vi "Make String.vi"(8 "error in (no error)":errorcluster, 11 "Construct String Setup Cam in":refnum<class "Construct String Setup Cam.lvclass">) -> (0 "error out":errorcluster, 2 "Camera Setup":string, 3 "Construct String Setup Cam out":refnum<class "Construct String Setup Cam.lvclass">)   [LabVIEW 2018, in "Construct String Setup Cam.lvclass"]
doc: "Este VI faz a leitura da configuração da câmera e constrói uma string com as informações da configuração."
uses:
  Construct String Setup Cam.lvclass
  Construct String Setup Cam.lvclass/Construct String Setup Cam.ctl
panel:
  out "Camera Setup 2":T1
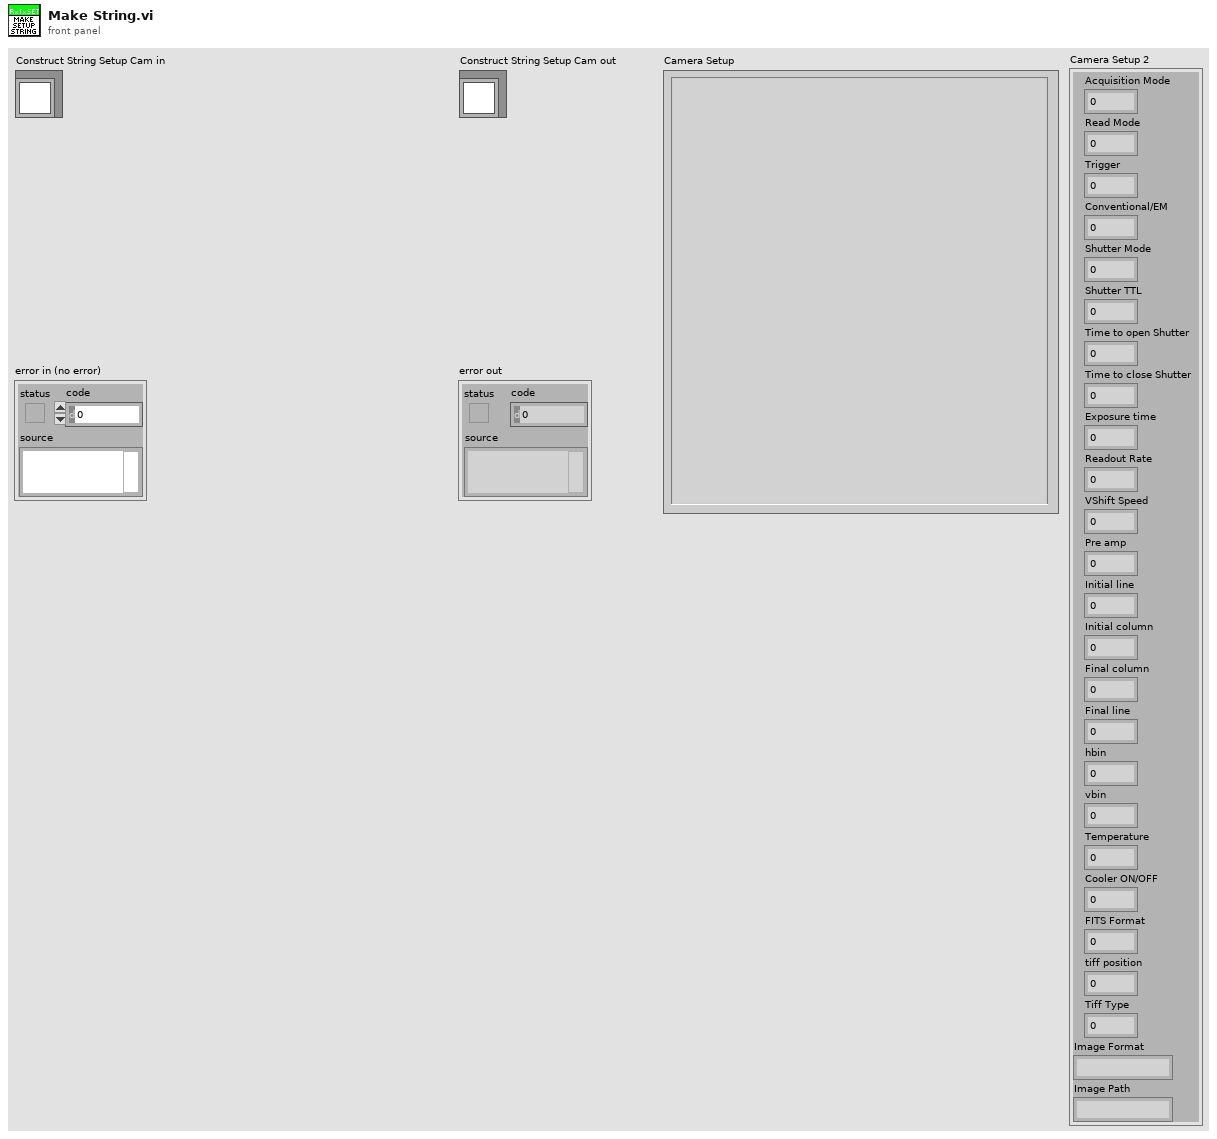
[diagram p1: front panel]
types:
  T1 = cluster{"Acquisition Mode":u16, "Read Mode":u16, "Trigger":u16, "Conventional/EM":u16, "Shutter Mode":u16, "Shutter TTL":u16, "Time to open Shutter":u16, "Time to close Shutter":u16, "Exposure time":dbl, "Readout Rate":u16, "VShift Speed":u16, "Pre amp":u16, "Initial line":u16, "Initial column":u16, "Final column":u32, "Final line":u32, "hbin":u16, "vbin":u16, "Temperature":dbl, "Cooler ON/OFF":u16, "FITS Format":u16, "tiff position":u16, "Tiff Type":u16, "Image Format":string, "Image Path":string}
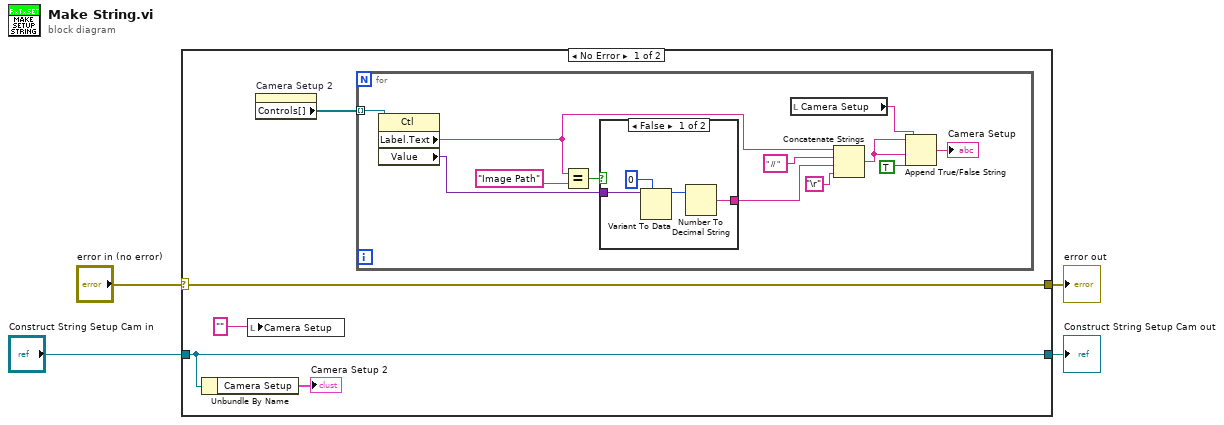
[diagram p0: block diagram]
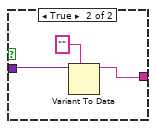
[diagram p2: hidden frame]
diagram:
  n1 = case shown="No Error" "error in (no error)" {
    selector: "error in (no error)" -> [w9 w30]
    tunnel: [w9 w30] -> w3
    tunnel: [w8 w29] -> w1
    tunnel: "Construct String Setup Cam in" -> [w8 w29]
    frame No Error {
      n2 = Unbundle By Name(w8) -> ("Camera Setup"=→"Camera Setup 2":T1)
      n3 = local write "Camera Setup"("") -> ()
      n4 = property on="Camera Setup 2" class="Clust (strict)"() -> ("Controls[]"=w5:refnum<vi>[])  [unwired: 2 in, 2 out]
      n5 = for {
        tunnel: w5 -> [w13] mode=indexing
        n6 = property on="Property Node" class="Ctl"(reference=w13) -> ("Label.Text"=w10:string, "Value"=w15:variant)  [unwired: 1 in, 2 out]
        n7 = Equal?(x=w10, y="Image Path") -> (x = y?=w12:bool)
        n8 = case shown="False" w12 {
          tunnel: w15 -> [w25 w27]
          tunnel: [w22 w26] -> w14
          frame False {
            n9 = Variant To Data(type=0, Variant=w25) -> (data=w23:i32)  [unwired: 1 in, 1 out]
            n10 = Number To Decimal String(number=w23) -> (decimal integer string=w22:string)  [unwired: 1 in]
          }
          frame True {
            n11 = Variant To Data(type="", Variant=w27) -> (data=w26:string)  [unwired: 1 in, 1 out]
          }
        }
        n12 = local read "Camera Setup"() -> (w20:string)
        n13 = Concatenate Strings(w10, " // ", w14, "\r") -> (w19:string)
        n14 = Append True/False String(1:TRUE ("selector"), 2:w19, 3:w19, 4:w20) -> (0:→"Camera Setup":string)
      }
    }
    frame Error {
    }
  }
  "error out" <- w3
  "Construct String Setup Cam out" <- w1
